vi "Autonomous Independent.vi"   [LabVIEW 2011]
doc: "This VI is called when autonomous begins, and will automatically be terminated when autonomous ends. You can carry out timed or sensor driven robot movement independently without needing to return to the caller."
uses:
  Robot Global Data.vi
types:
  T1 = typedef "WPI_DigitalInputDevRef.ctl" = cluster{"DevStatus":errorcluster, "DIO Channel":T2, "Digital Module":T3}
  T2 = typedef "FPGA_DIOChannel.ctl" = enum8{"DIO 1", "DIO 2", "DIO 3", "DIO 4", "DIO 5", "DIO 6", "DIO 7", "DIO 8", "DIO 9", "DIO 10", "DIO 11", "DIO 12", "DIO 13", "DIO 14", "Invalid"}
  T3 = typedef "FPGA_TypedefDigitalModule.ctl" = enum16{"Digital Module 1", "Digital Module 2"}
  T4 = typedef "WPI_MotorControlDeviceRef.ctl" = cluster{"DeviceStatus":errorcluster, "Type":enum16{"PWM", "CAN"}, "PWM":cluster{"Digital Module":T3, "PWM Channel":T5, "DeadBand":T6}, "CAN":cluster{"Device Number":u8, "Control Mode":T7, "Semaphore":T8, "Max Vout":dbl}, "Invert":bool, "TransformRef":T9, "InvTransformRef":T9}
  T5 = typedef "FPGA_DIOPWMChannel.ctl" = enum8{"PWM 1", "PWM 2", "PWM 3", "PWM 4", "PWM 5", "PWM 6", "PWM 7", "PWM 8", "PWM 9", "PWM 10", "Invalid"}
  T6 = typedef "WPI_PWMDeadband.ctl" = cluster{"Name":string, "maxPositivePwm":i32, "minPositivePwm":i32, "centerPwm":i32, "maxNegativePwm":i32, "minNegativePwm":i32, "angularRange":u16}
  T7 = typedef "WPI_CANJaguar_ControlMode.ctl" = enum8{"Percent VBus", "Current", "Speed", "Position", "Voltage"}
  T8 = typedef "Semaphore RefNum" = refnum<k1>
  T9 = typedef "WPI_PWMTransform_ConPane.ctl" = refnum<vi>
  T10 = typedef "WPI_JoystickDevRef.ctl" = cluster{"Device":T11}
  T11 = typedef "WPI_JoystickDeviceEnum.ctl" = enum16{"USB 1", "USB 2", "USB 3", "USB 4", "Kinect 1", "Kinect 2"}
  T12 = cluster{"axis 1 (x)":dbl, "axis 2 (y)":dbl, "axis 3 (throttle)":dbl, "axis 4":dbl, "axis 5":dbl, "axis 6":dbl}
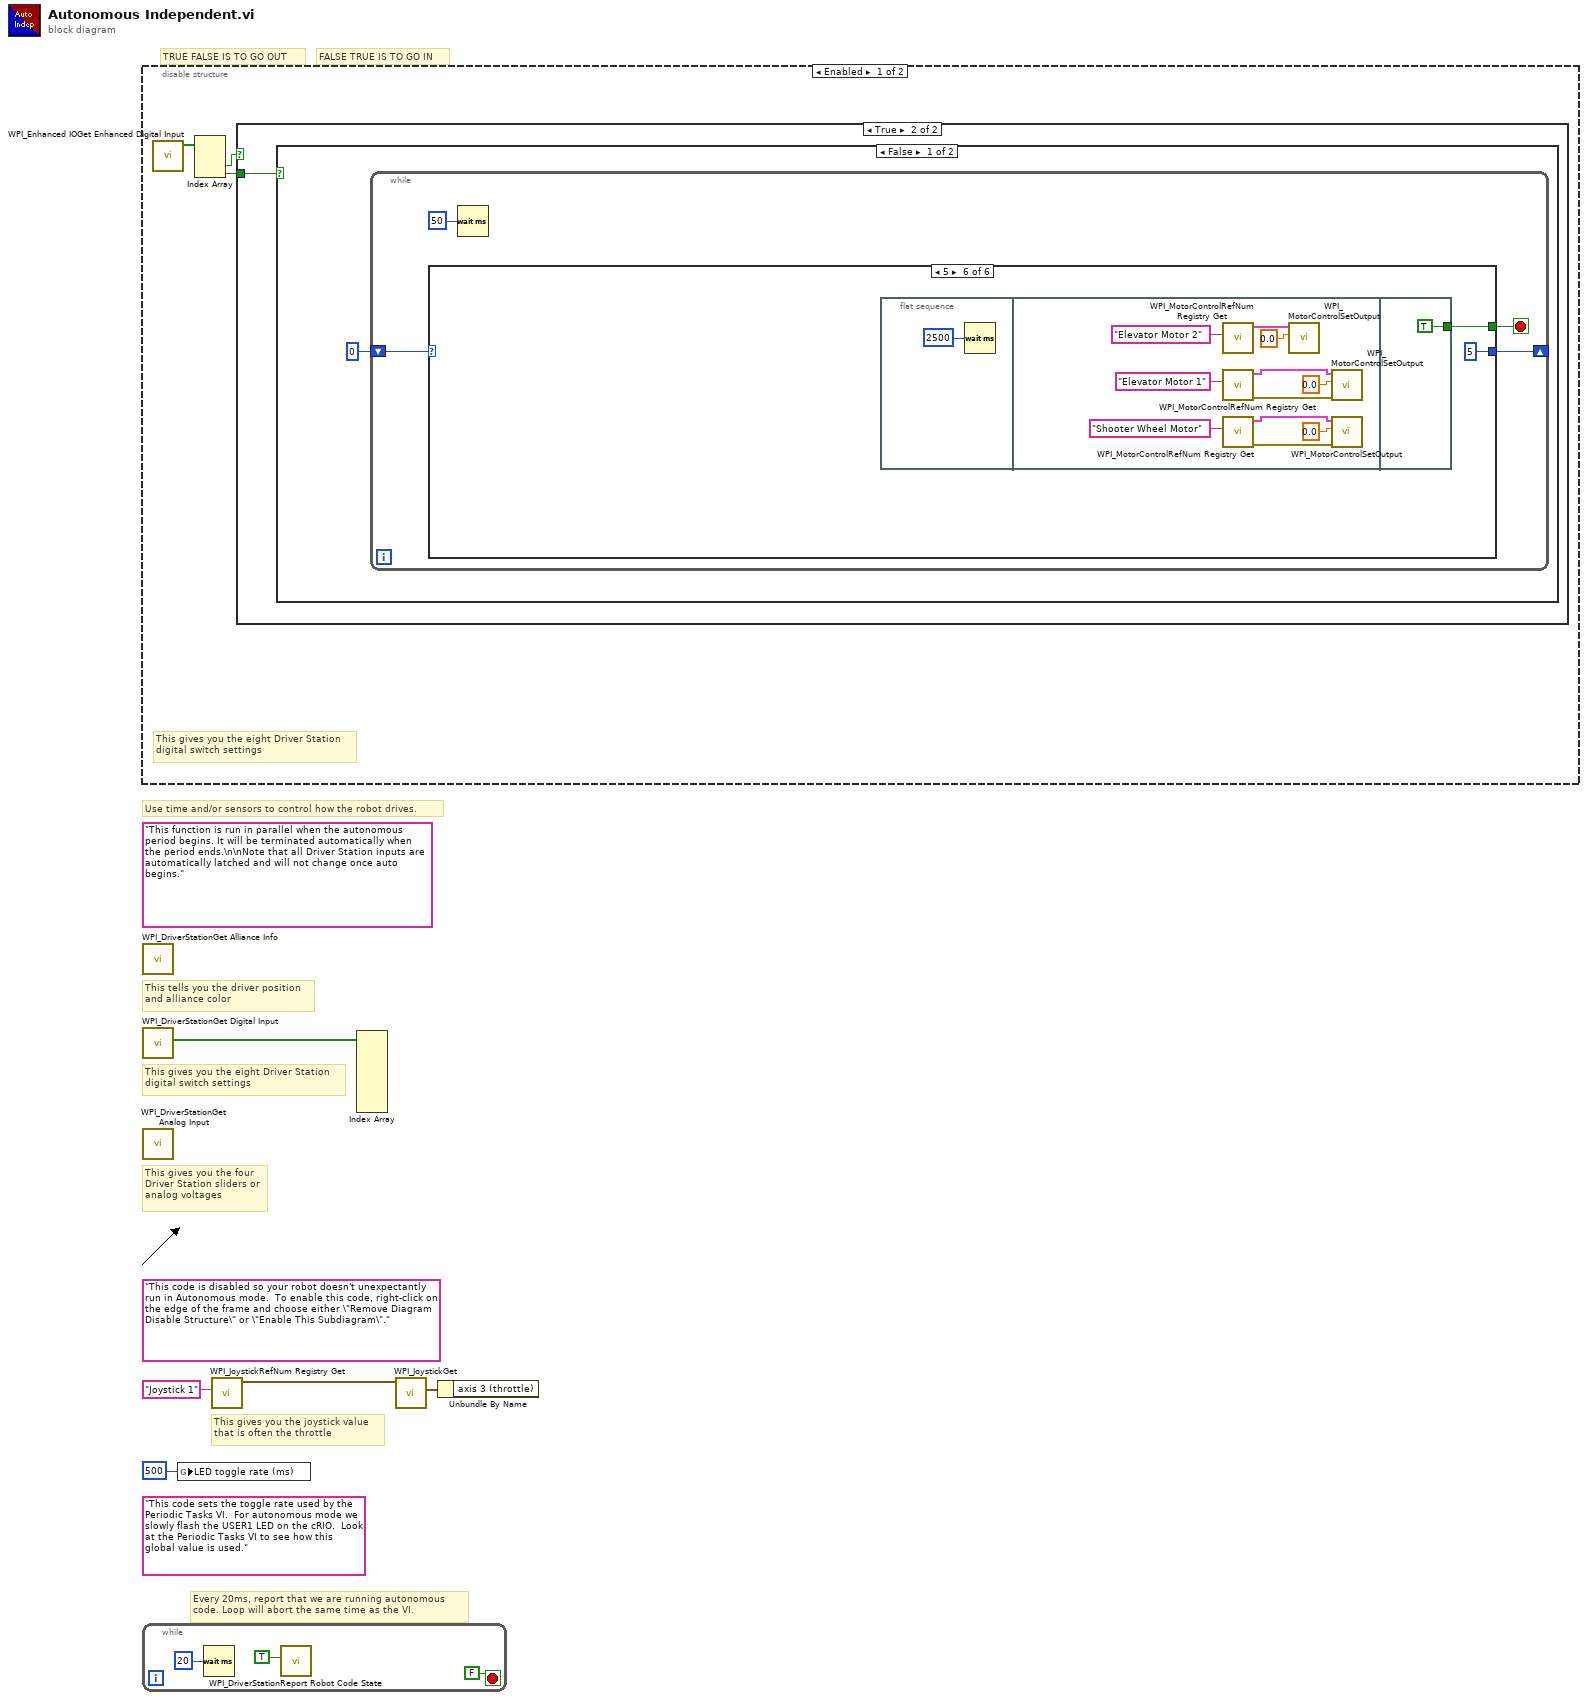
[diagram p0: block diagram]
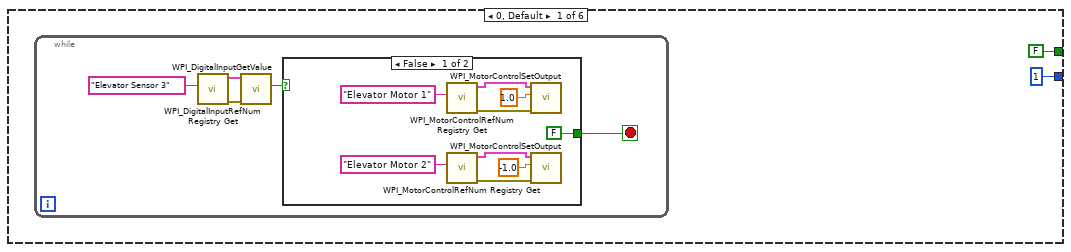
[diagram p4: hidden frame]
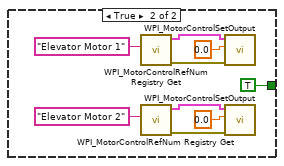
[diagram p5: hidden frame]
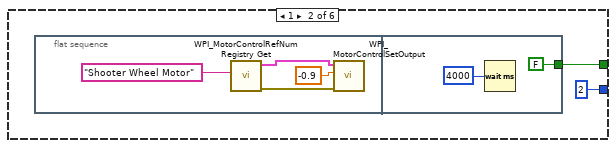
[diagram p6: hidden frame]
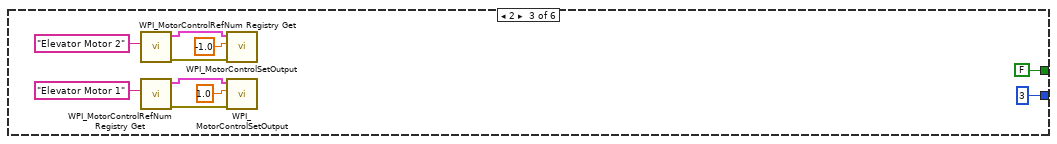
[diagram p7: hidden frame]
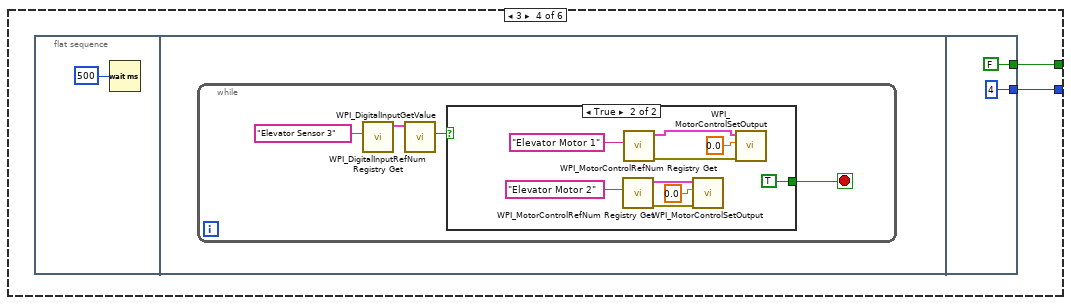
[diagram p8: hidden frame]
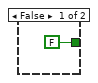
[diagram p9: hidden frame]
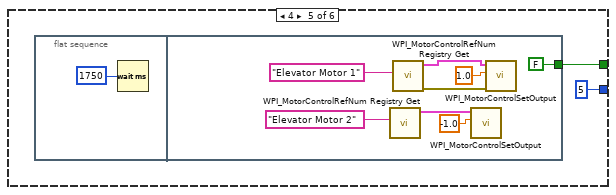
[diagram p10: hidden frame]
diagram:
  (unwired) "This code sets the toggle rate used by the Periodic Tasks VI.  For autonomous mode we slowly flash the USER1 LED on the cRIO.  Look at the Periodic Tasks VI to see how this global value is used."
  (unwired) "This code is disabled so your robot doesn't unexpectantly run in Autonomous mode.  To enable this code, right-click on the edge of the frame and choose either \"Remove Diagram Disable Structure\" or \"Enable This Subdiagram\"."
  (unwired) "This function is run in parallel when the autonomous period begins. It will be terminated automatically when the period ends.\n\nNote that all Driver Station inputs are automatically latched and will not change once auto begins."
  # "FALSE TRUE IS TO GO IN"
  # "TRUE FALSE IS TO GO OUT"
  # "Every 20ms, report that we are running autonomous\ncode. Loop will abort the same time as the VI."
  # "This gives you the joystick value\nthat is often the throttle"
  # "Use time and/or sensors to control how the robot drives."
  # "This tells you the driver position\nand alliance color"
  # "This gives you the eight Driver Station\ndigital switch settings"
  # "This gives you the four\nDriver Station sliders or\nanalog voltages"
  n1 = disable-structure shown="Enabled" {
    frame Enabled {
      # "This gives you the eight Driver Station\ndigital switch settings"
      n2 = call <vilib>:"WPI_Enhanced IOGet Enhanced Digital Input.vi"() -> ("Digital Input [1-16]"=w8:bool[])  [unwired: 10 in, 1 out]
      n3 = Index Array(array=w8) -> (element #2=w7:bool, element #3=w6:bool)  [unwired: 3 in, 1 out]
      n4 = case shown="True" w7 {
        tunnel: w6 -> [w9 w10]
        frame False {
          n5 = case shown="True" w9 {
            frame False {
            }
            frame True {
              # "Encoders AUTO"
            }
          }
        }
        frame True {
          n6 = case shown="False" w10 {
            frame False {
              n7 = while {
                shift-right: [w13] -> _
                shift-left: 0 -> [w12]
                stop <- w14 stop-if-true
                n8 = case shown="5" w12 {
                  tunnel: [1 2 3 w59 5 5] -> w13
                  tunnel: [FALSE w41 FALSE w60 w78 w89] -> w14
                  frame 0, Default {
                    n9 = while {
                      stop <- w22 stop-if-true
                      n10 = call <vilib>:"WPI_DigitalInputRefNum Registry Get.vi"("refnum name"="Elevator Sensor 3") -> ("error out"=w21:errorcluster, "DigitalInputDevRef"=w20:T1)  [unwired: 9 in]
                      n11 = call <vilib>:"WPI_DigitalInputGetValue.vi"("error in (no error)"=w21, "DigitalInputDevRef"=w20) -> ("Value"=w18:bool)  [unwired: 7 in, 2 out]
                      n12 = case shown="False" w18 {
                        tunnel: [FALSE TRUE] -> w22
                        frame False {
                          n13 = call <vilib>:"WPI_MotorControlRefNum Registry Get.vi"("refnum name"="Elevator Motor 1") -> ("error out"=w28:errorcluster, "MotorControlDevRef"=w27:T4)  [unwired: 9 in]
                          n14 = call <vilib>:"WPI_MotorControlRefNum Registry Get.vi"("refnum name"="Elevator Motor 2") -> ("error out"=w31:errorcluster, "MotorControlDevRef"=w24:T4)  [unwired: 9 in]
                          n15 = call <vilib>:"WPI_MotorControlSetOutput.vi"("error in (no error)"=w28, "Output"=1.0, "MotorControlDevRef"=w27) -> ()  [unwired: 7 in, 2 out]
                          n16 = call <vilib>:"WPI_MotorControlSetOutput.vi"("error in (no error)"=w31, "Output"=-1.0, "MotorControlDevRef"=w24) -> ()  [unwired: 7 in, 2 out]
                        }
                        frame True {
                          n17 = call <vilib>:"WPI_MotorControlRefNum Registry Get.vi"("refnum name"="Elevator Motor 1") -> ("error out"=w37:errorcluster, "MotorControlDevRef"=w36:T4)  [unwired: 9 in]
                          n18 = call <vilib>:"WPI_MotorControlRefNum Registry Get.vi"("refnum name"="Elevator Motor 2") -> ("error out"=w40:errorcluster, "MotorControlDevRef"=w33:T4)  [unwired: 9 in]
                          n19 = call <vilib>:"WPI_MotorControlSetOutput.vi"("error in (no error)"=w37, "Output"=0.0, "MotorControlDevRef"=w36) -> ()  [unwired: 7 in, 2 out]
                          n20 = call <vilib>:"WPI_MotorControlSetOutput.vi"("error in (no error)"=w40, "Output"=0.0, "MotorControlDevRef"=w33) -> ()  [unwired: 7 in, 2 out]
                        }
                      }
                    }
                  }
                  frame 1 {
                    n21 = flat-sequence {
                      tunnel: [FALSE] -> w41
                      frame #0 {
                        n22 = call <vilib>:"WPI_MotorControlRefNum Registry Get.vi"("refnum name"="Shooter Wheel Motor") -> ("error out"=w46:errorcluster, "MotorControlDevRef"=w43:T4)  [unwired: 9 in]
                        n23 = call <vilib>:"WPI_MotorControlSetOutput.vi"("error in (no error)"=w46, "Output"=-0.9, "MotorControlDevRef"=w43) -> ()  [unwired: 7 in, 2 out]
                      }
                      frame #1 {
                        n24 = Wait (ms)(milliseconds to wait=u32 4000) -> ()  [unwired: 1 out]
                      }
                    }
                  }
                  frame 2 {
                    n25 = call <vilib>:"WPI_MotorControlRefNum Registry Get.vi"("refnum name"="Elevator Motor 2") -> ("error out"=w49:errorcluster, "MotorControlDevRef"=w50:T4)  [unwired: 9 in]
                    n26 = call <vilib>:"WPI_MotorControlRefNum Registry Get.vi"("refnum name"="Elevator Motor 1") -> ("error out"=w53:errorcluster, "MotorControlDevRef"=w54:T4)  [unwired: 9 in]
                    n27 = call <vilib>:"WPI_MotorControlSetOutput.vi"("error in (no error)"=w49, "Output"=-1.0, "MotorControlDevRef"=w50) -> ()  [unwired: 7 in, 2 out]
                    n28 = call <vilib>:"WPI_MotorControlSetOutput.vi"("error in (no error)"=w53, "Output"=1.0, "MotorControlDevRef"=w54) -> ()  [unwired: 7 in, 2 out]
                  }
                  frame 3 {
                    n29 = flat-sequence {
                      tunnel: [FALSE] -> w60
                      tunnel: [4] -> w59
                      frame #0 {
                        n30 = Wait (ms)(milliseconds to wait=u32 500) -> ()  [unwired: 1 out]
                      }
                      frame #1 {
                        n31 = while {
                          stop <- w62 stop-if-true
                          n32 = call <vilib>:"WPI_DigitalInputRefNum Registry Get.vi"("refnum name"="Elevator Sensor 3") -> ("DigitalInputDevRef"=w64:T1)  [unwired: 9 in, 1 out]
                          n33 = call <vilib>:"WPI_DigitalInputGetValue.vi"("DigitalInputDevRef"=w64) -> ("Value"=w63:bool)  [unwired: 8 in, 2 out]
                          n34 = case shown="True" w63 {
                            tunnel: [FALSE TRUE] -> w62
                            frame False {
                            }
                            frame True {
                              n35 = call <vilib>:"WPI_MotorControlRefNum Registry Get.vi"("refnum name"="Elevator Motor 2") -> ("error out"=w67:errorcluster, "MotorControlDevRef"=w69:T4)  [unwired: 9 in]
                              n36 = call <vilib>:"WPI_MotorControlRefNum Registry Get.vi"("refnum name"="Elevator Motor 1") -> ("error out"=w70:errorcluster, "MotorControlDevRef"=w71:T4)  [unwired: 9 in]
                              n37 = call <vilib>:"WPI_MotorControlSetOutput.vi"("error in (no error)"=w67, "Output"=0.0, "MotorControlDevRef"=w69) -> ()  [unwired: 7 in, 2 out]
                              n38 = call <vilib>:"WPI_MotorControlSetOutput.vi"("error in (no error)"=w70, "Output"=0.0, "MotorControlDevRef"=w71) -> ()  [unwired: 7 in, 2 out]
                            }
                          }
                        }
                      }
                      frame #2 {
                      }
                    }
                  }
                  frame 4 {
                    n39 = flat-sequence {
                      tunnel: [FALSE] -> w78
                      frame #0 {
                        n40 = Wait (ms)(milliseconds to wait=u32 1750) -> ()  [unwired: 1 out]
                      }
                      frame #1 {
                        n41 = call <vilib>:"WPI_MotorControlRefNum Registry Get.vi"("refnum name"="Elevator Motor 2") -> ("MotorControlDevRef"=w88:T4)  [unwired: 9 in, 1 out]
                        n42 = call <vilib>:"WPI_MotorControlRefNum Registry Get.vi"("refnum name"="Elevator Motor 1") -> ("error out"=w87:errorcluster, "MotorControlDevRef"=w81:T4)  [unwired: 9 in]
                        n43 = call <vilib>:"WPI_MotorControlSetOutput.vi"("Output"=-1.0, "MotorControlDevRef"=w88) -> ()  [unwired: 8 in, 2 out]
                        n44 = call <vilib>:"WPI_MotorControlSetOutput.vi"("error in (no error)"=w87, "Output"=1.0, "MotorControlDevRef"=w81) -> ()  [unwired: 7 in, 2 out]
                      }
                    }
                  }
                  frame 5 {
                    n45 = flat-sequence {
                      tunnel: [TRUE] -> w89
                      frame #0 {
                        n46 = Wait (ms)(milliseconds to wait=u32 2500) -> ()  [unwired: 1 out]
                      }
                      frame #1 {
                        n47 = call <vilib>:"WPI_MotorControlRefNum Registry Get.vi"("refnum name"="Elevator Motor 2") -> ("MotorControlDevRef"=w98:T4)  [unwired: 9 in, 1 out]
                        n48 = call <vilib>:"WPI_MotorControlRefNum Registry Get.vi"("refnum name"="Elevator Motor 1") -> ("error out"=w97:errorcluster, "MotorControlDevRef"=w92:T4)  [unwired: 9 in]
                        n49 = call <vilib>:"WPI_MotorControlRefNum Registry Get.vi"("refnum name"="Shooter Wheel Motor") -> ("error out"=w102:errorcluster, "MotorControlDevRef"=w99:T4)  [unwired: 9 in]
                        n50 = call <vilib>:"WPI_MotorControlSetOutput.vi"("Output"=0.0, "MotorControlDevRef"=w98) -> ()  [unwired: 8 in, 2 out]
                        n51 = call <vilib>:"WPI_MotorControlSetOutput.vi"("error in (no error)"=w97, "Output"=0.0, "MotorControlDevRef"=w92) -> ()  [unwired: 7 in, 2 out]
                        n52 = call <vilib>:"WPI_MotorControlSetOutput.vi"("error in (no error)"=w102, "Output"=0.0, "MotorControlDevRef"=w99) -> ()  [unwired: 7 in, 2 out]
                      }
                      frame #2 {
                      }
                    }
                  }
                }
                n53 = Wait (ms)(milliseconds to wait=u32 50) -> ()  [unwired: 1 out]
              }
            }
            frame True {
            }
          }
        }
      }
    }
    frame Disabled {
    }
  }
  n54 = call <vilib>:"WPI_DriverStationGet Alliance Info.vi"() -> ()  [unwired: 12 out]
  n55 = call <vilib>:"WPI_DriverStationGet Digital Input.vi"() -> ("Driver Station Digital Input (1-8)"=w5:bool[])  [unwired: 11 out]
  n56 = call <vilib>:"WPI_DriverStationGet Analog Input.vi"() -> ()  [unwired: 12 out]
  n57 = while {
    stop <- FALSE stop-if-true
    n58 = Wait (ms)(milliseconds to wait=u32 20) -> ()  [unwired: 1 out]
    n59 = call <vilib>:"WPI_DriverStationReport Robot Code State.vi"("Autonomous"=TRUE) -> ()  [unwired: 10 in, 1 out]
  }
  n60 = global write "Robot Global Data.vi" "LED toggle rate (ms)"(u32 500 ("LED ms toggle rate")) -> ()
  n61 = call <vilib>:"WPI_JoystickRefNum Registry Get.vi"("refnum name"="Joystick 1") -> ("JoystickDevRef"=w2:T10)  [unwired: 1 in, 9 out]
  n62 = Index Array(array=w5) -> ()  [unwired: 8 in, 8 out]
  n63 = call <vilib>:"WPI_JoystickGet.vi"("JoystickDevRef"=w2) -> ("Axes"=w3:T12)  [unwired: 1 in, 5 out]
  n64 = Unbundle By Name(w3) -> ()  [unwired: 1 out]
